vi "reprTextual.vi"(8 "error in (no error)":errorcluster, 11 "Drive in":refnum<class "Drive.lvclass">) -> (0 "error out":errorcluster, 2 "Description":string, 3 "Drive out":refnum<class "Drive.lvclass">)   [LabVIEW 2011, in "Drive.lvclass"]
uses:
  Drive.lvclass
  Drive.lvclass/Drive.ctl
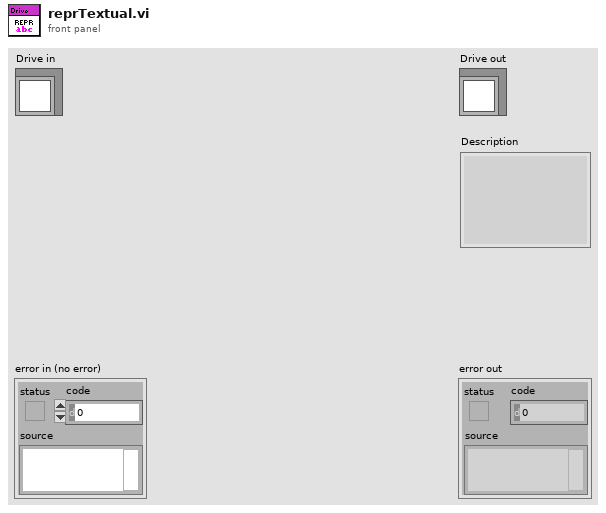
[diagram p1: front panel]
types:
  T1 = typedef "UTM Location.ctl" = cluster{"UTM Zone":dbl, "Hemisphere":enum16{"North", "South"}, "East":dbl, "North":dbl}
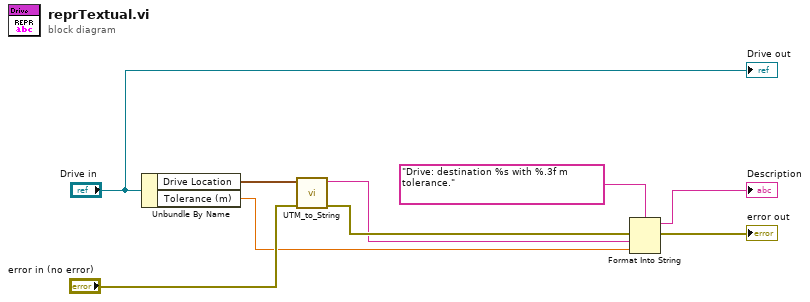
[diagram p0: block diagram]
diagram:
  n1 = Unbundle By Name("Drive in") -> ("Drive Location"=w7:T1, "Tolerance (m)"=w2:dbl)
  n2 = call "UTM_to_String.vi"("error in"="error in (no error)", "UTM Location"=w7) -> ("error out"=w5:errorcluster, "UTM String"=w1:string)  [unwired: 8 in]
  n3 = Format Into String(format string="Drive: destination %s with %.3f m tolerance.", error in=w5, w1, w2) -> (resulting string=→"Description":string, error out=→"error out":errorcluster)  [unwired: 1 in]
  "Drive out" <- "Drive in"
